vi "Taiko_SimpleDemo.vi"() -> ()   [LabVIEW 2010]
uses:
  _lib/PDLM/pdlm_lib_x86_x64_UIThread.llb/PDLM_SystemStatus.ctl
  _lib/PDLM/pdlm_lib_x86_x64_UIThread.llb/PDLM_LaserMode.ctl
  _lib/PDLM/pdlm_lib_x86_x64_UIThread.llb/PDLM_LHData_LaserType.ctl
  _lib/PDLM/pdlm_lib_x86_x64_UIThread.llb/PDLM_LHVersion.ctl
  _lib/PDLM/pdlm_lib_x86_x64_UIThread.llb/PDLM_LHData.ctl
  _lib/PDLM/pdlm_lib_x86_x64_UIThread.llb/PDLM_Tag.ctl
  _lib/PDLM/pdlm_lib_x86_x64_UIThread.llb/PDLM_DllPath_global.vi
  _lib/PDLM/pdlm_lib_x86_x64_UIThread.llb/PDLM_TaggedValueList.ctl
  _lib/PDLM/pdlm_lib_x86_x64_UIThread.llb/PDLM_TaggedValue.ctl
panel:
  out "Errror":errorcluster
  in  "Exit":bool
  in  "Update":bool
  out "String":string
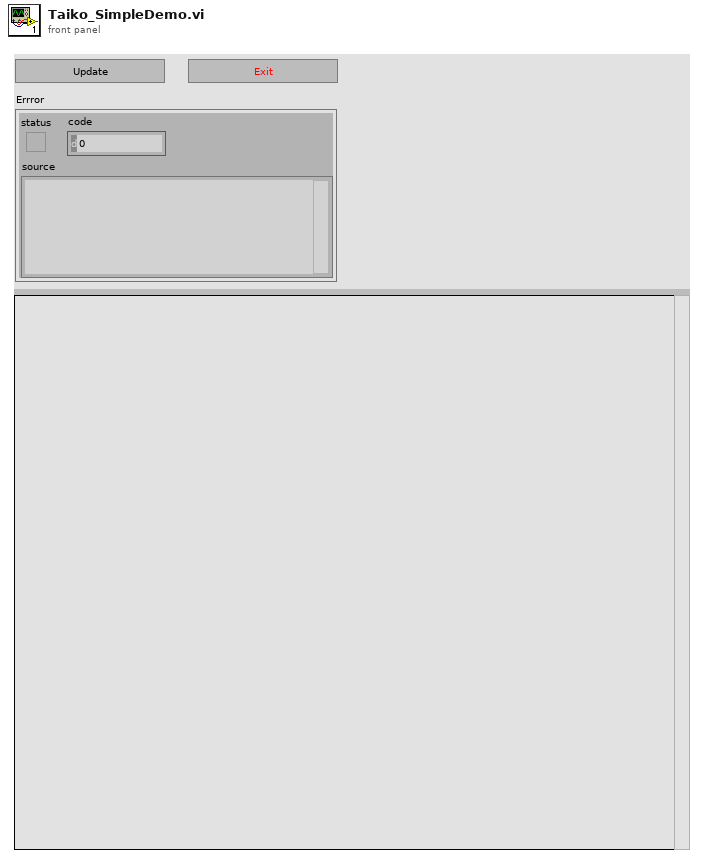
[diagram p1: front panel]
types:
  T1 = typedef "PDLM_LHData.ctl" = cluster{"SerNo":u32, "Features":u32, "FreqMin":u32, "FreqMax":u32, "CwPowerMax":u32, "PulsePowerMax":u32, "WavelengthNominal":u16, "CaseTempMax":u16, "Protection":bool, "LHTypeCtrlVoltage":u16, "LHMaxVoltage":u16, "CurrentTEP12V":u16, "LaserType":T2, "LHVersion":T3, "CalWarrentHours":u16}
  T2 = typedef "PDLM_LHData_LaserType.ctl" = u16
  T3 = typedef "PDLM_LHVersion.ctl" = cluster{"Major":u16, "Minor":u16}
  T4 = typedef "PDLM_LaserMode.ctl" = enum32{"CW", "PULSE", "BURST"}
  T5 = typedef "PDLM_TaggedValueList.ctl" = T6[]
  T6 = typedef "PDLM_TaggedValue.ctl" = cluster{"Tag":T7, "Value":u32}
  T7 = typedef "PDLM_Tag.ctl" = u32
  T8 = typedef "PDLM_SystemStatus.ctl" = u32
  T9 = typedef "PDLM_LHInfo.ctl" = cluster{"LType":string, "Date":string, "LClass":string}
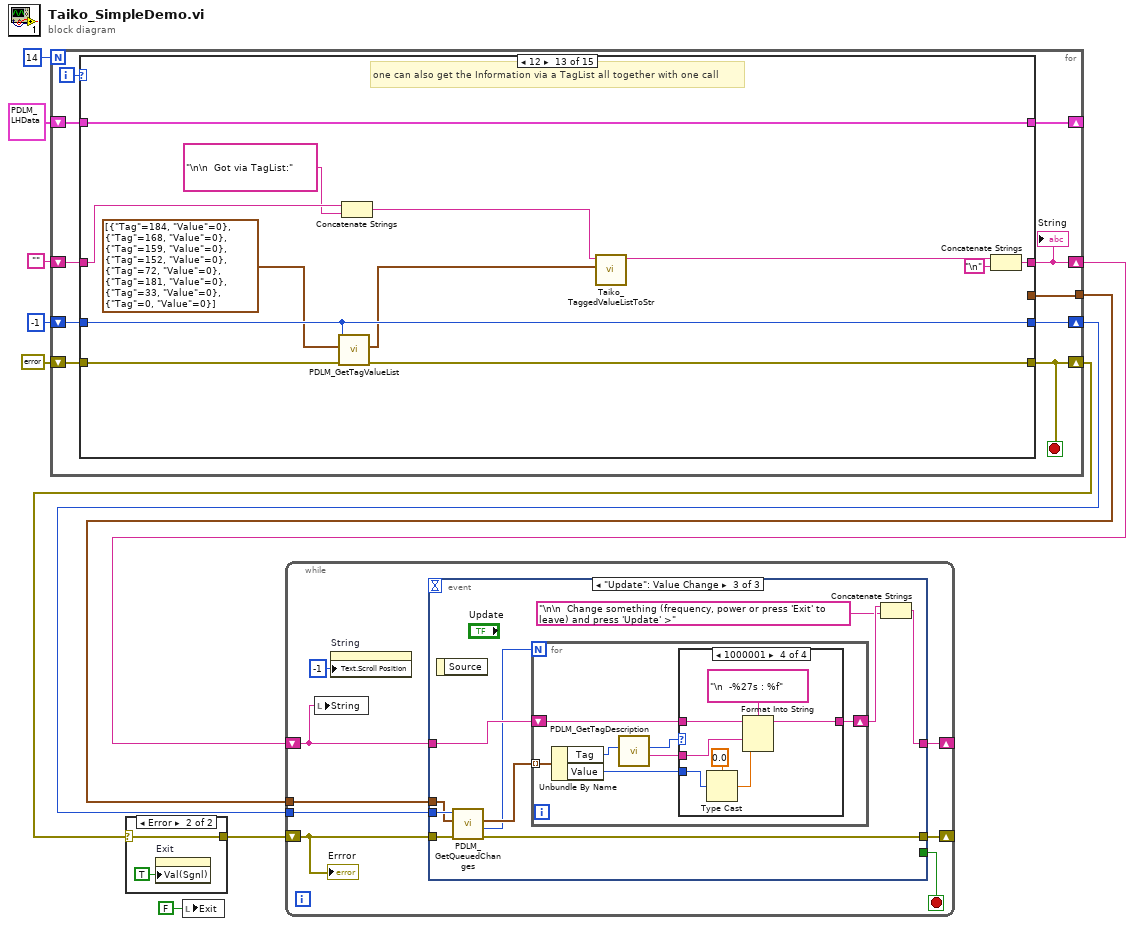
[diagram p0: block diagram]
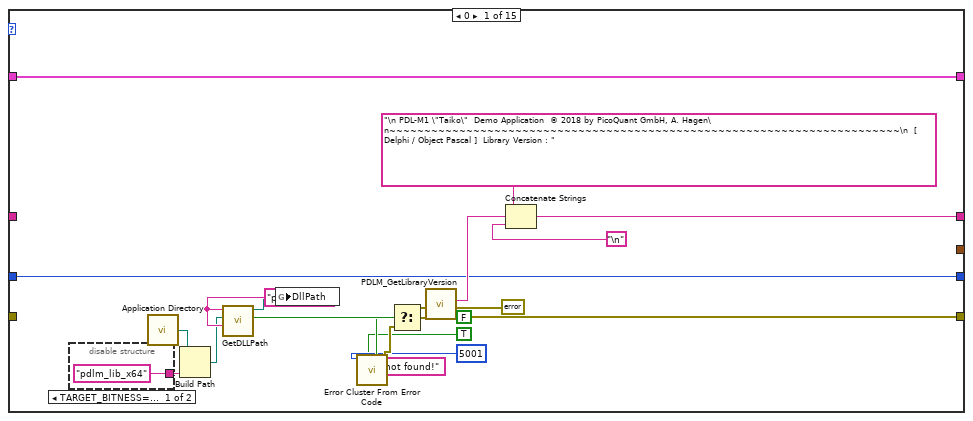
[diagram p3: hidden frame]
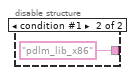
[diagram p4: hidden frame]
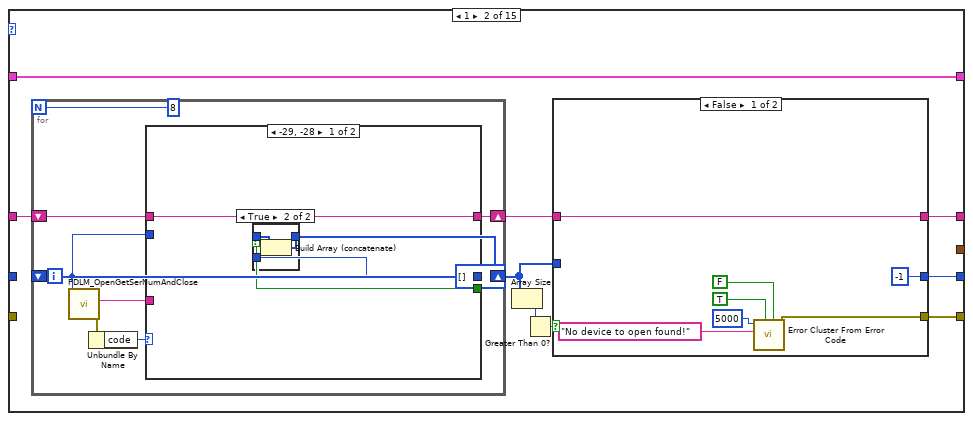
[diagram p5: hidden frame]
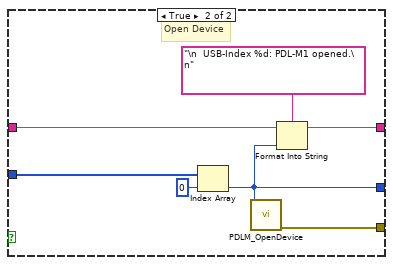
[diagram p6: hidden frame]
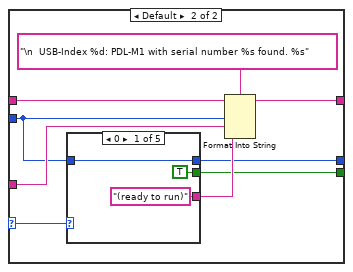
[diagram p8: hidden frame]
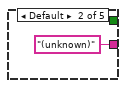
[diagram p9: hidden frame]
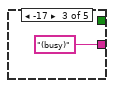
[diagram p10: hidden frame]
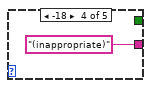
[diagram p11: hidden frame]
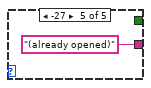
[diagram p12: hidden frame]
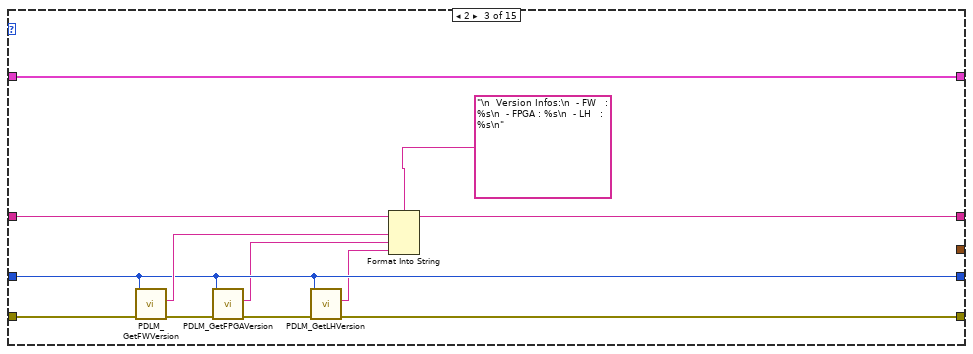
[diagram p13: hidden frame]
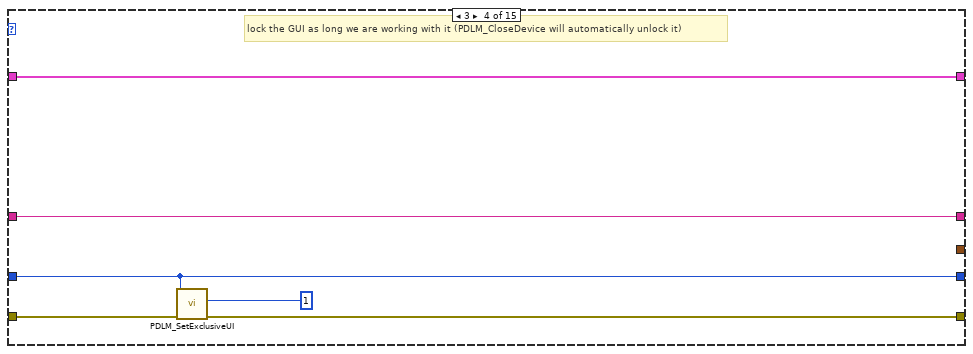
[diagram p14: hidden frame]
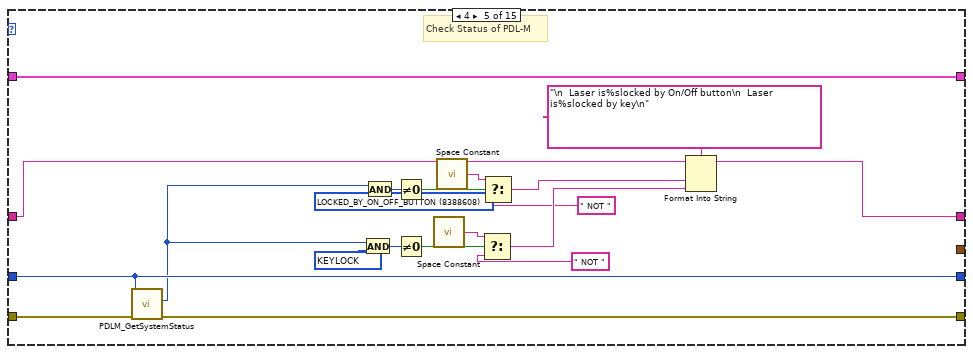
[diagram p15: hidden frame]
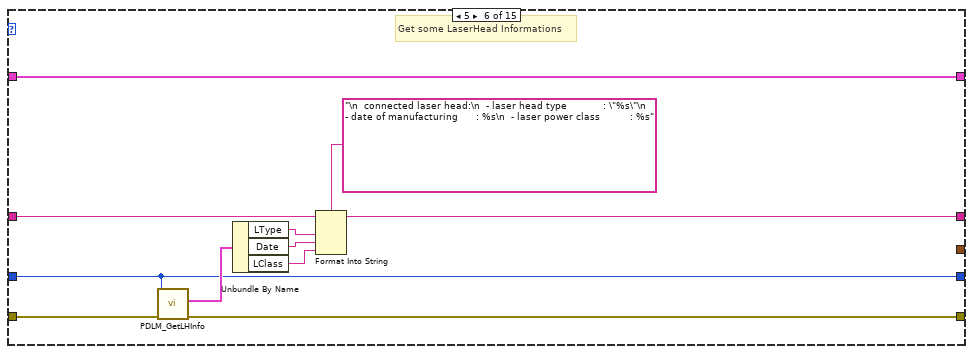
[diagram p16: hidden frame]
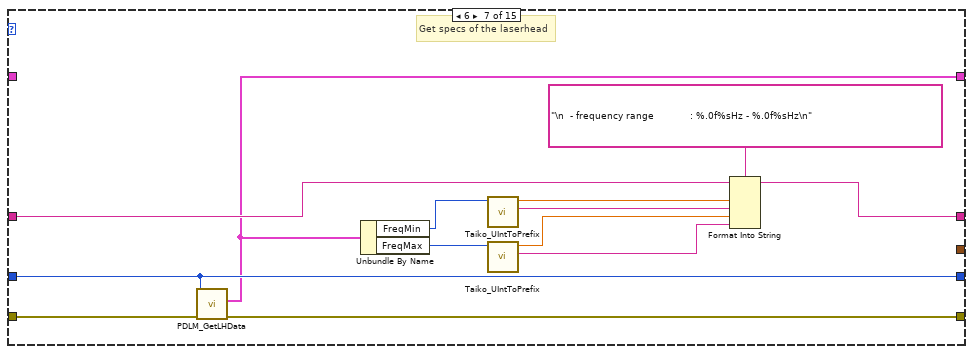
[diagram p17: hidden frame]
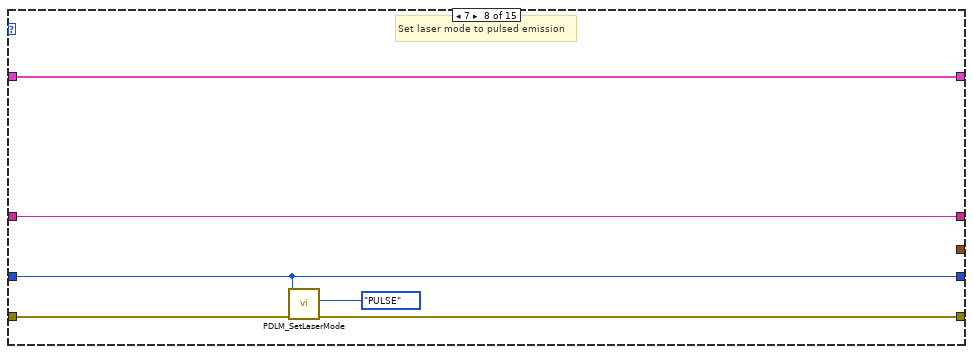
[diagram p18: hidden frame]
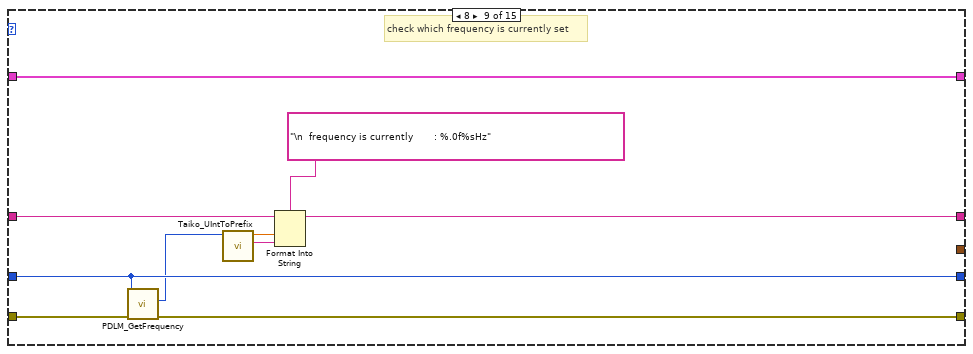
[diagram p19: hidden frame]
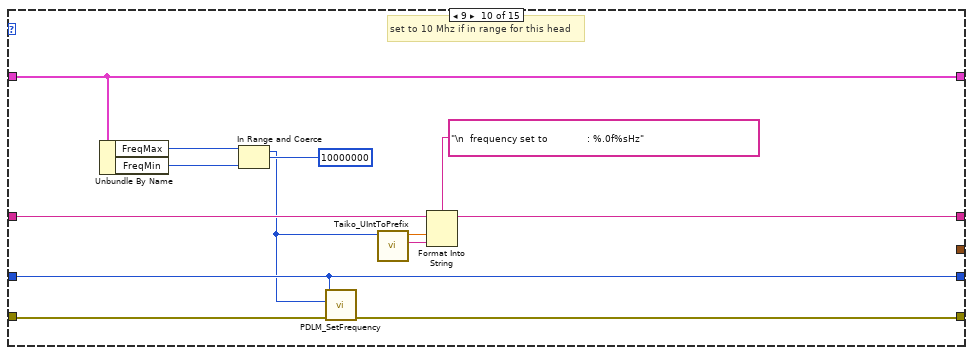
[diagram p20: hidden frame]
diagram:
  n1 = for {
    N: 14 -> [_]
    shift-right: [w15] -> w5
    shift-left: "" -> [w17]
    shift-right: [w16] -> w3
    shift-left: errorcluster {"status"=FALSE, "code"=0, "source"=""} ("error out") -> [w20]
    shift-right: [w18] -> w6
    shift-left: -1 -> [w19]
    shift-right: [w14] -> _
    shift-left: T1 {"SerNo"=0, "Features"=0, "FreqMin"=0, "FreqMax"=0, "CwPowerMax"=0, "PulsePowerMax"=0, "WavelengthNominal"=0, "CaseTempMax"=0, "Protection"=FALSE, "LHTypeCtrlVoltage"=0, "LHMaxVoltage"=0, "CurrentTEP12V"=0, "LaserType"=0, "LHVersion"={"Major"=0, "Minor"=0}, "CalWarrentHours"=0} ("Data") -> [w13]
    tunnel: [w12] -> w4
    i -> [w21]
    stop <- w16 stop-if-true
    n2 = case shown="12" w21 {
      tunnel: [w39 w47 w107 w113 w124 w139 w156 w163 w172 w182 w192 w201 w211 w223 w235] -> w15
      tunnel: [w38 w48 w101 w115 w136 w143 w159 w165 w175 w185 w194 w205 w216 w226 w237] -> w16
      tunnel: w20 -> [_ _ w111 w116 w137 w144 w160 w166 w176 w186 w195 w206 w217 w230 w237]
      tunnel: w19 -> [w37 _ w104 w114 w135 w142 w158 w164 w174 w184 w193 w200 w215 w225 w236]
      tunnel: [w37 w49 w104 w114 w135 w142 w158 w164 w174 w184 w193 w200 w215 w225 w236] -> w18
      tunnel: w17 -> [_ w53 w109 w113 w125 w140 w157 w163 w173 w183 w192 w202 w208 w224 w235]
      tunnel: [w35 w45 w100 w112 w122 w138 w155 w162 w171 w190 w191 w204 w218 w229 w234] -> w14
      tunnel: w13 -> [w35 w45 w100 w112 w122 w138 _ w162 w171 w190 w191 w204 w218 w229 w234]
      tunnel: [_ _ _ _ _ _ _ _ _ _ _ _ _ w219 _] -> w12
      frame 0 {
        w34 = "pdlm_lib.dll" ("DllName_64bit")
        n3 = disable-structure shown="TARGET_BITNESS==64, Default" {
          disable-tunnel: ["pdlm_lib_x64" "pdlm_lib_x86"] -> w32
          frame condition #0 (active) {
          }
          frame condition #1 {
          }
        }
        n4 = call <vilib>:"Application Directory.vi"() -> ("Application Directory"=w33:path)
        n5 = Build Path(base path=w33, name or relative path=w32) -> (appended path=w31:path)
        n6 = call "GetDLLPath.vi"("DllName_32bit"=w34, "PathToDLL"=w31, "DllName_64bit"=w34) -> ("file exists?"=w29:bool, "DLLPath"=w30:path)  [unwired: 7 in]
        n7 = global write "PDLM_DllPath_global.vi" "DllPath"(w30) -> ()
        n8 = call <vilib>:"Error Cluster From Error Code.vi"("is warning? (False)"=FALSE, "show call chain? (False)"=TRUE, "error message (\"\")"="DLL not found!" ("error message (\"\")"), "error code (0)"=5001) -> ("error out"=w26:errorcluster)  [unwired: 5 in]
        n9 = Select(t=errorcluster {"status"=FALSE, "code"=0, "source"=""} ("error in (no error)"), s=w29, f=w26) -> (s? t:f=w27:errorcluster)
        n10 = call "PDLM_GetLibraryVersion.vi"("error in (no error)"=w27) -> ("error out"=w38:errorcluster, "Version"=w41:string)  [unwired: 8 in, 1 out]
        n11 = Concatenate Strings("\n PDL-M1 \"Taiko\"  Demo Application  © 2018 by PicoQuant GmbH, A. Hagen\n~~~~~~~~~~~~~~~~~~~~~~~~~~~~~~~~~~~~~~~~~~~~~~~~~~~~~~~~~~~~~~~~~~~~~~~~~\n  [ Delphi / Object Pascal ]  Library Version : ", w41, "\n") -> (w39:string)
      }
      frame 1 {
        n12 = for {
          N: 8 -> [_]
          shift-right: [w75] -> w46
          shift-left: w53 -> [w76]
          shift-right: [w69] -> w50
          shift-left: i32[] [] ("Array") -> [w70]
          i -> [w74]
          n13 = call "PDLM_OpenGetSerNumAndClose.vi"("USBIdx"=w74) -> ("error out"=w77:errorcluster, "SerNo"=w78:string)  [unwired: 8 in, 1 out]
          n14 = Unbundle By Name(w77) -> ("code"=w71:i32)
          n15 = case shown="-29, -28" w71 {
            selector: w71 -> [_ w84]
            tunnel: w78 -> [_ w92]
            tunnel: w76 -> [w83 w89]
            tunnel: [w83 w88] -> w75
            tunnel: w74 -> [_ w87]
            tunnel: [_ w86] -> w73
            tunnel: [_ w85] -> w72
            frame -29, -28 {
            }
            frame Default {
              n16 = case shown="0" w84 {
                tunnel: ["(ready to run)" "(unknown)" "(busy)" "(inappropriate)" "(already opened)"] -> w91
                tunnel: w87 -> [w94 _ _ _ _]
                tunnel: [w94 _ _ _ _] -> w86
                tunnel: [TRUE _ _ _ _] -> w85
                frame 0 {
                }
                frame Default {
                }
                frame -17 {
                }
                frame -18 {
                }
                frame -27 {
                }
              }
              n17 = Format Into String(format string="\n  USB-Index %d: PDL-M1 with serial number %s found. %s", initial string=w89, w87, w92, w91) -> (resulting string=w88:string)  [unwired: 1 in, 1 out]
            }
          }
          n18 = case shown="True" w72 {
            tunnel: w70 -> [w79 w81]
            tunnel: w73 -> [_ w80]
            tunnel: [w79 w82] -> w69
            frame False {
            }
            frame True {
              n19 = Build Array (concatenate)(w81, w80) -> (w82:i32[])
            }
          }
        }
        n20 = Array Size(array=w50) -> (size(s)=w52:i32)
        n21 = Greater Than 0?(x=w52) -> (x > 0?=w51:bool)
        n22 = case shown="False" w51 {
          tunnel: w50 -> [_ w68]
          tunnel: [-1 w63] -> w49
          tunnel: [w60 w66] -> w48
          tunnel: [w59 w64] -> w47
          tunnel: w46 -> [w59 w65]
          frame False {
            n23 = call <vilib>:"Error Cluster From Error Code.vi"("is warning? (False)"=FALSE, "show call chain? (False)"=TRUE, "error message (\"\")"="No device to open found!" ("error message (\"\")"), "error code (0)"=5000) -> ("error out"=w60:errorcluster)  [unwired: 5 in]
          }
          frame True {
            # "Open Device"
            n24 = Index Array(array=w68, index=0) -> (element=w63:i32)
            n25 = call "PDLM_OpenDevice.vi"("USBIdx"=w63) -> ("error out"=w66:errorcluster)  [unwired: 8 in, 2 out]
            n26 = Format Into String(format string="\n  USB-Index %d: PDL-M1 opened.\n", initial string=w65, w63) -> (resulting string=w64:string)  [unwired: 1 in, 1 out]
          }
        }
      }
      frame 2 {
        n27 = call "PDLM_GetFWVersion.vi"("error in (no error)"=w111, "USBIdx"=w104) -> ("error out"=w106:errorcluster, "Version"=w110:string)  [unwired: 7 in, 1 out]
        n28 = call "PDLM_GetFPGAVersion.vi"("error in (no error)"=w106, "USBIdx"=w104) -> ("error out"=w105:errorcluster, "Version"=w103:string)  [unwired: 7 in, 1 out]
        n29 = call "PDLM_GetLHVersion.vi"("error in (no error)"=w105, "USBIdx"=w104) -> ("error out"=w101:errorcluster, "Version"=w102:string)  [unwired: 7 in, 1 out]
        n30 = Format Into String(format string="\n  Version Infos:\n  - FW   : %s\n  - FPGA : %s\n  - LH   : %s\n", initial string=w109, w110, w103, w102) -> (resulting string=w107:string)  [unwired: 1 in, 1 out]
      }
      frame 3 {
        # "lock the GUI as long we are working with it (PDLM_CloseDevice will automatically unlock it)"
        n31 = call "PDLM_SetExclusiveUI.vi"("error in (no error)"=w116, "mode"=u32 1, "USBIdx"=w114) -> ("error out"=w115:errorcluster)  [unwired: 7 in, 1 out]
      }
      frame 4 {
        w130 = T8 33554432 items=["INITIALIZING"=1, "DEVICE_UNCALIBRATED"=2, "COMMISSIONING_MODE"=4, "LASERHEAD_SAFETY_MODE"=8, "FW_UPDATE_RUNNING"=16, "DEVICE_DEFECT"=32, "DEVICE_INCOMPATIBLE"=64, "BUSY"=128, "EXCLUSIVE_SW_OP_GRANTED"=256, "PARAMETER_CHANGES_PENDING"=512, "LASERHEAD_CHANGED"=2048, "LASERHEAD_MISSING"=4096, "LASERHEAD_DEFECT"=8192, "LASERHEAD_UNKNOWN_TYPE"=16384, "LASERHEAD_DECALIBRATED"=32768, "LASERHEAD_DIODE_TEMP_TOO_LOW"=65536, "LASERHEAD_DIODE_TEMP_TOO_HIGH"=131072, "LASERHEAD_DIODE_OVERHEATING"=262144, "LASERHEAD_CASE_OVERHEATING"=524288, "LASERHEAD_FAN_RUNNING"=1048576, "LASERHEAD_INCOMPATIBLE"=2097152, "LOCKED_BY_EXPIRED_DEMO_MODE"=4194304, "LOCKED_BY_ON_OFF_BUTTON"=8388608, "SOFTLOCK"=16777216, "KEYLOCK"=33554432, "LOCKED_BY_SECURITY_POLICY"=67108864, "INTERLOCK"=134217728, "LASERHEAD_PULSE_POWER_INACCURATE"=268435456, "ERRORMSG_PENDING"=2147483648] ("SystemStatus")
        w129 = T8 8388608 items=["INITIALIZING"=1, "DEVICE_UNCALIBRATED"=2, "COMMISSIONING_MODE"=4, "LASERHEAD_SAFETY_MODE"=8, "FW_UPDATE_RUNNING"=16, "DEVICE_DEFECT"=32, "DEVICE_INCOMPATIBLE"=64, "BUSY"=128, "EXCLUSIVE_SW_OP_GRANTED"=256, "PARAMETER_CHANGES_PENDING"=512, "LASERHEAD_CHANGED"=2048, "LASERHEAD_MISSING"=4096, "LASERHEAD_DEFECT"=8192, "LASERHEAD_UNKNOWN_TYPE"=16384, "LASERHEAD_DECALIBRATED"=32768, "LASERHEAD_DIODE_TEMP_TOO_LOW"=65536, "LASERHEAD_DIODE_TEMP_TOO_HIGH"=131072, "LASERHEAD_DIODE_OVERHEATING"=262144, "LASERHEAD_CASE_OVERHEATING"=524288, "LASERHEAD_FAN_RUNNING"=1048576, "LASERHEAD_INCOMPATIBLE"=2097152, "LOCKED_BY_EXPIRED_DEMO_MODE"=4194304, "LOCKED_BY_ON_OFF_BUTTON"=8388608, "SOFTLOCK"=16777216, "KEYLOCK"=33554432, "LOCKED_BY_SECURITY_POLICY"=67108864, "INTERLOCK"=134217728, "LASERHEAD_PULSE_POWER_INACCURATE"=268435456, "ERRORMSG_PENDING"=2147483648] ("SystemStatus")
        # "Check Status of PDL-M"
        n32 = call "PDLM_GetSystemStatus.vi"("error in (no error)"=w137, "USBIdx"=w135) -> ("error out"=w136:errorcluster, "state"=w128:u32)  [unwired: 7 in, 1 out]
        n33 = And(x=w128, y=w130) -> (x .and. y?=w132:T8)
        n34 = And(x=w128, y=w129) -> (x .and. y?=w131:T8)
        n35 = Not Equal To 0?(x=w131) -> (x != 0?=w133:bool)
        n36 = Not Equal To 0?(x=w132) -> (x != 0?=w134:bool)
        n37 = call <vilib>:"Space Constant.vi"() -> ("String"=w121:string)
        n38 = call <vilib>:"Space Constant.vi"() -> ("String"=w119:string)
        n39 = Select(t=w121, s=w134, f=" NOT ") -> (s? t:f=w126:string)
        n40 = Select(t=w119, s=w133, f=" NOT ") -> (s? t:f=w127:string)
        n41 = Format Into String(format string="\n  Laser is%slocked by On/Off button\n  Laser is%slocked by key\n", initial string=w125, w127, w126) -> (resulting string=w124:string)  [unwired: 1 in, 1 out]
      }
      frame 5 {
        # "Get some LaserHead Informations"
        n42 = call "PDLM_GetLHInfo.vi"("error in (no error)"=w144, "USBIdx"=w142) -> ("error out"=w143:errorcluster, "LHInfo"=w145:T9)  [unwired: 7 in, 1 out]
        n43 = Unbundle By Name(w145) -> ("LType"=w146:string, "Date"=w147:string, "LClass"=w148:string)
        n44 = Format Into String(format string="\n  connected laser head:\n  - laser head type            : \"%s\"\n  - date of manufacturing      : %s\n  - laser power class          : %s", initial string=w140, w146, w147, w148) -> (resulting string=w139:string)  [unwired: 1 in, 1 out]
      }
      frame 6 {
        # "Get specs of the laserhead"
        n45 = call "PDLM_GetLHData.vi"("error in (no error)"=w160, "USBIdx"=w158) -> ("error out"=w159:errorcluster, "Data"=w155:T1)  [unwired: 7 in, 1 out]
        n46 = Unbundle By Name(w155) -> ("FreqMin"=w151:u32, "FreqMax"=w154:u32)
        n47 = call "Taiko_UIntToPrefix.vi"("UINT"=w151) -> ("PREFIX"=w149:string, "MANT"=w150:sgl)  [unwired: 9 in]
        n48 = call "Taiko_UIntToPrefix.vi"("UINT"=w154) -> ("PREFIX"=w152:string, "MANT"=w153:sgl)  [unwired: 9 in]
        n49 = Format Into String(format string="\n  - frequency range            : %.0f%sHz - %.0f%sHz\n", initial string=w157, w150, w149, w153, w152) -> (resulting string=w156:string)  [unwired: 1 in, 1 out]
      }
      frame 7 {
        # "Set laser mode to pulsed emission"
        n50 = call "PDLM_SetLaserMode.vi"("error in (no error)"=w166, "mode"=PDLM_LaserMode."PULSE", "USBIdx"=w164) -> ("error out"=w165:errorcluster)  [unwired: 7 in, 1 out]
      }
      frame 8 {
        # "check which frequency is currently set"
        n51 = call "PDLM_GetFrequency.vi"("error in (no error)"=w176, "USBIdx"=w174) -> ("error out"=w175:errorcluster, "freq"=w170:u32)  [unwired: 7 in, 1 out]
        n52 = call "Taiko_UIntToPrefix.vi"("UINT"=w170) -> ("PREFIX"=w168:string, "MANT"=w169:sgl)  [unwired: 9 in]
        n53 = Format Into String(format string="\n  frequency is currently       : %.0f%sHz", initial string=w173, w169, w168) -> (resulting string=w172:string)  [unwired: 1 in, 1 out]
      }
      frame 9 {
        # "set to 10 Mhz if in range for this head"
        n54 = Unbundle By Name(w190) -> ("FreqMax"=w189:u32, "FreqMin"=w188:u32)
        n55 = In Range and Coerce(upper limit=w189, x=u32 10000000 ("freq"), lower limit=w188) -> (coerced(x)=w180:u32)  [unwired: 1 out]
        n56 = call "PDLM_SetFrequency.vi"("error in (no error)"=w186, "freq"=w180, "USBIdx"=w184) -> ("error out"=w185:errorcluster)  [unwired: 7 in, 1 out]
        n57 = call "Taiko_UIntToPrefix.vi"("UINT"=w180) -> ("PREFIX"=w178:string, "MANT"=w179:sgl)  [unwired: 9 in]
        n58 = Format Into String(format string="\n  frequency set to             : %.0f%sHz", initial string=w183, w179, w178) -> (resulting string=w182:string)  [unwired: 1 in, 1 out]
      }
      frame 10 {
        # "Set Power"
        n59 = call "PDLM_SetPulsePowerPermille.vi"("error in (no error)"=w195, "permille"=u32 50, "USBIdx"=w193) -> ("error out"=w194:errorcluster)  [unwired: 7 in, 1 out]
      }
      frame 11 {
        # "read the resulting Power in mW"
        n60 = call "PDLM_GetPulsePower.vi"("error in (no error)"=w206, "USBIdx"=w200) -> ("error out"=w205:errorcluster, "Power"=w199:sgl)  [unwired: 7 in, 1 out]
        n61 = call "Taiko_SGLToPrefix.vi"("SGL"=w199) -> ("PREFIX"=w197:string, "MANT"=w198:sgl)  [unwired: 9 in]
        n62 = Format Into String(format string="\n  pulse power set to           : %.3f%sW", initial string=w202, w198, w197) -> (resulting string=w201:string)  [unwired: 1 in, 1 out]
      }
      frame 12 {
        # "one can also get the Information via a TagList all together with one call"
        n63 = call "PDLM_GetTagValueList.vi"("error in (no error)"=w217, "TaggedValueList"=T5 [{"Tag"=184, "Value"=0}, {"Tag"=168, "Value"=0}, {"Tag"=159, "Value"=0}, {"Tag"=152, "Value"=0}, {"Tag"=72, "Value"=0}, {"Tag"=181, "Value"=0}, {"Tag"=33, "Value"=0}, {"Tag"=0, "Value"=0}], "USBIdx"=w215) -> ("error out"=w216:errorcluster, "TaggedValueList out"=w213:T5)  [unwired: 6 in, 1 out]
        n64 = Concatenate Strings(w208, "\n\n  Got via TagList:" ("string")) -> (w209:string)
        n65 = call "Taiko_TaggedValueListToStr.vi"("TaggedValueList in"=w213, "String in"=w209) -> ("String out"=w212:string)  [unwired: 9 in]
        n66 = Concatenate Strings(w212, "\n") -> (w211:string)
      }
      frame 13 {
        # "Unlock the Device GUI and ask user to change something"
        n67 = call "PDLM_SetExclusiveUI.vi"("error in (no error)"=w230, "mode"=u32 0, "USBIdx"=w225) -> ("error out"=w228:errorcluster)  [unwired: 7 in, 1 out]
        n68 = flat-sequence {
          tunnel: w228 -> [w232]
          tunnel: [w232] -> w227
          frame #0 {
            n69 = Wait (ms)(milliseconds to wait=u32 100) -> ()  [unwired: 1 out]
          }
        }
        n70 = Initialize Array(cluster{"Tag":T7, "Value":u32} {"Tag"=0, "Value"=0} ("TaggedValue"), 50 ("dimension size")) -> (w219:cluster{"Tag":T7, "Value":u32}[])
        n71 = call "PDLM_GetQueuedChanges.vi"("error in (no error)"=w227, "TaggedValueList"=w219, "USBIdx"=w225) -> ("error out"=w226:errorcluster)  [unwired: 5 in, 3 out]
        n72 = Concatenate Strings(w224, "\n  Device GUI unlocked\n\n\n  Change something (frequency, power or press 'Exit' to leave) and press 'Update' >" ("string")) -> (w223:string)
      }
      frame Default {
      }
    }
    "String" <- w15
  }
  n73 = case shown="Error" w3 {
    selector: w3 -> [w238 w240]
    tunnel: [w238 w240] -> w2
    frame No Error {
    }
    frame Error {
      n74 = property on="Exit" class="Bool (strict)"("Val(Sgnl)"=TRUE ("Value (Signaling)")) -> ()  [unwired: 2 in, 2 out]
    }
  }
  n75 = local write "Exit"(FALSE ("Exit")) -> ()
  n76 = while {
    tunnel: w6 -> [w247]
    tunnel: w4 -> [w246]
    shift-right: [w245] -> _
    shift-left: w5 -> [w242]
    shift-right: [w244] -> _
    shift-left: w2 -> [w243]
    stop <- w248 stop-if-true
    n77 = local write "String"(w242) -> ()
    n78 = property on="String" class="Str"("Text.Scroll Position"=-1) -> ()  [unwired: 2 in, 2 out]
    n79 = event shown="[2] \"Update\": Value Change" {
      selector: _ -> [_ _ _]
      dyn-events: _ -> [_ _ _]
      timeout: _ -> [_ _ _]
      tunnel: [TRUE TRUE _] -> w248
      tunnel: w247 -> [w251 w255 w266]
      tunnel: w242 -> [w250 w253 w262]
      tunnel: w246 -> [_ _ w265]
      tunnel: [w250 w253 w257] -> w245
      tunnel: w243 -> [_ _ w264]
      tunnel: [w249 _ w263] -> w244
      event "Exit": Value Change {
        n80 = event-data() -> ()  [unwired: 1 in, 6 out]
        n81 = call "PDLM_CloseDevice.vi"("USBIdx"=w251) -> ("error out"=w249:errorcluster)  [unwired: 9 in, 1 out]
      }
      event Panel Close? {
        n82 = event-data() -> ()  [unwired: 1 in, 1 out]
        n83 = call "PDLM_CloseDevice.vi"("USBIdx"=w255) -> ()  [unwired: 9 in, 2 out]
        n84 = event-data("Discard?"=TRUE) -> ()  [unwired: 1 in, 1 out]
      }
      event "Update": Value Change {
        n85 = event-data() -> ()  [unwired: 1 in, 1 out]
        n86 = call "PDLM_GetQueuedChanges.vi"("error in (no error)"=w264, "TaggedValueList"=w265, "USBIdx"=w266) -> ("error out"=w263:errorcluster, "ListLen out"=w260:u32, "TaggedValueList out"=w261:T5)  [unwired: 5 in, 1 out]
        n87 = for {
          N: w260 -> [_]
          tunnel: w261 -> [w273] mode=indexing
          shift-right: [w269] -> w259
          shift-left: w262 -> [w268]
          n88 = Unbundle By Name(w273) -> ("Tag"=w272:T7, "Value"=w270:u32)
          n89 = call "PDLM_GetTagDescription.vi"("Tag"=w272) -> ("Name"=w271:string, "TypeCode"=w267:u32)  [unwired: 7 in, 2 out]
          n90 = case shown="1000001" w267 {
            tunnel: w271 -> [_ w279 w286 w293]
            tunnel: w270 -> [_ w277 w281 w288]
            tunnel: [w274 w276 w284 w291] -> w269
            tunnel: w268 -> [w274 w275 w283 w290]
            frame Default {
            }
            frame 1..69377 {
              n91 = Format Into String(format string="\n  -%27s : %d", initial string=w275, w279, w277) -> (resulting string=w276:string)  [unwired: 1 in, 1 out]
            }
            frame 1114113..16777215 {
              n92 = Type Cast(type=0, x=w281) -> (*(type *) &x=w280:i32)
              n93 = Format Into String(format string="\n  -%27s : %d", initial string=w283, w286, w280) -> (resulting string=w284:string)  [unwired: 1 in, 1 out]
            }
            frame 16777217 {
              n94 = Type Cast(type=sgl 0.0, x=w288) -> (*(type *) &x=w287:sgl)
              n95 = Format Into String(format string="\n  -%27s : %f", initial string=w290, w293, w287) -> (resulting string=w291:string)  [unwired: 1 in, 1 out]
            }
          }
        }
        n96 = Concatenate Strings(w259, "\n\n  Change something (frequency, power or press 'Exit' to leave) and press 'Update' >") -> (w257:string)
      }
    }
    "Errror" <- w243
  }
